vi "Status-string.vi"(11 "Duration [s]":dbl) -> (3 "String":string)   [LabVIEW 2013, in "PowderDeposition.lvlib" / "Move-Timer.lvclass"]
uses:
  Move-Timer.lvclass
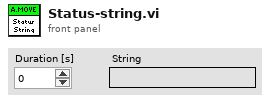
[diagram p1: front panel]
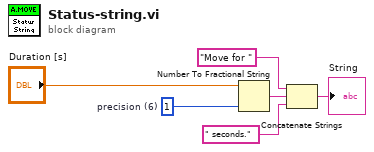
[diagram p0: block diagram]
diagram:
  w6 = i16 1  # precision (6)
  n1 = Number To Fractional String(number="Duration [s]", precision (6)=w6) -> (F-format string=w1:string)  [unwired: 2 in]
  n2 = Concatenate Strings("Move for ", w1, " seconds.") -> (→"String":string)
